vi "GetModuleNames.vi"(11 "moduleName":string) -> (1 "module":string, 2 "angle":string, 3 "drive":string)   [LabVIEW 2020]
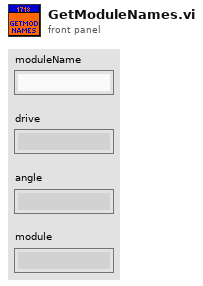
[diagram p1: front panel]
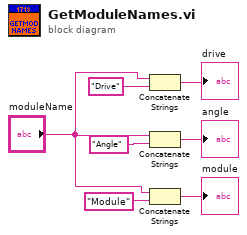
[diagram p0: block diagram]
diagram:
  n1 = Concatenate Strings("moduleName", "Drive" ("string")) -> (→"drive":string)
  n2 = Concatenate Strings("moduleName", "Angle" ("string")) -> (→"angle":string)
  n3 = Concatenate Strings("moduleName", "Module" ("string")) -> (→"module":string)
